vi "Set VLIW Array.vi"(8 "error in (no error)":errorcluster, 10 "VLIW Array":T1(array[cluster]), 11 "Slave_Pulseblaster in":refnum<class "Slave_Pulseblaster.lvclass">) -> (0 "error out":errorcluster, 3 "Slave_Pulseblaster out":refnum<class "Slave_Pulseblaster.lvclass">)   [LabVIEW 2013, in "Slave_Pulseblaster.lvclass"]
uses:
  Slave_Pulseblaster.lvclass
  Slave_Pulseblaster.lvclass/Slave_Pulseblaster.ctl
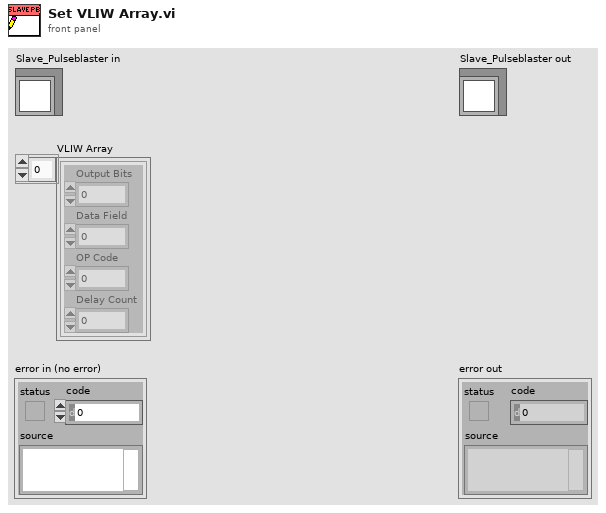
[diagram p1: front panel]
types:
  T1 = cluster{"Output Bits":u32, "Data Field":u32, "OP Code":u8, "Delay Count":u64}[]
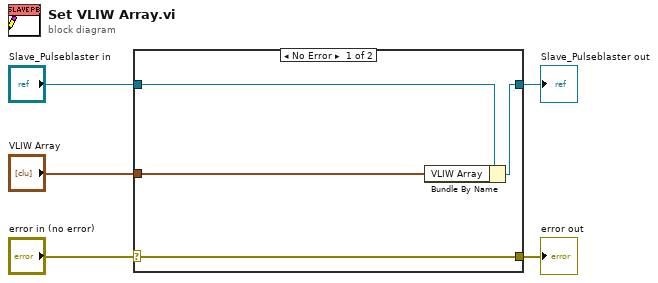
[diagram p0: block diagram]
diagram:
  n1 = case shown="No Error" "error in (no error)" {
    selector: "error in (no error)" -> [w9 w10]
    tunnel: [w9 w10] -> w4
    tunnel: [w7 w11] -> w2
    tunnel: "Slave_Pulseblaster in" -> [w8 w11]
    tunnel: "VLIW Array" -> [w6 _]
    frame No Error {
      n2 = Bundle By Name(cluster=w8, "VLIW Array"=w6) -> (w7:refnum<class "Slave_Pulseblaster.lvclass">)
    }
    frame Error {
    }
  }
  "error out" <- w4
  "Slave_Pulseblaster out" <- w2
